vi "AVS_SetParameter.vi"(0 "a_hDevice":i32, 7 "a_pDeviceParm":u8[](array[numeric])) -> (4 "Output Value":i32, 8 "a_pDeviceParm":u8[](array[numeric]))   [LabVIEW 2020]
uses:
  AvaSpecX64-DLL_9.4/avaspecx64.dll
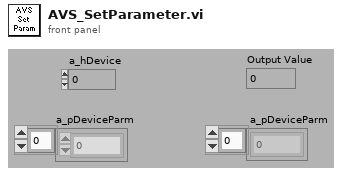
[diagram p1: front panel]
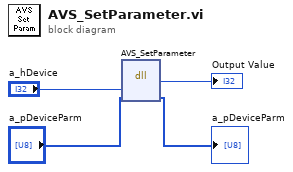
[diagram p0: block diagram]
diagram:
  n1 = dll-call lib="C:/AvaSpecX64-DLL_9.4/avaspecx64.dll" fn="AVS_SetParameter"("a_hDevice"="a_hDevice", "a_pDeviceParm"="a_pDeviceParm") -> ("return type"=→"Output Value":i32, "a_pDeviceParm"=→"a_pDeviceParm":u8[])  [unwired: 4 in, 2 out]
